vi "BNO055 Read Eular Example.vi"() -> ()   [LabVIEW 2019]
uses:
  <vilib>/myRIO/Common/Instrument Driver Framework/myRIO v1.0/UART/vis/myRIO v1.0 Close UART.vi
  <vilib>/myRIO/Common/Instrument Driver Framework/Utilities/vis/FPGA Ref Manager.vi
  <vilib>/myRIO/Common/Instrument Driver Framework/myRIO v1.0/myRIO v1.0 Reset FPGA.vi
  <vilib>/myRIO/Common/Instrument Driver Framework/myRIO v1.0/IRQ/vis/myRIO v1.0 IRQ Info FGV.vi
  <vilib>/myRIO/Common/Instrument Driver Framework/myRIO v1.0/IRQ/vis/myRIO v1.0 Timer IRQ Info FGV.vi
  <vilib>/myRIO/Common/Instrument Driver Framework/myRIO v1.0/IRQ/vis/myRIO v1.0 ISR Agent.vi
  <vilib>/myRIO/Instrument Drivers/Utilities/vis/Reset Index.vi
  <vilib>/myRIO/Common/Instrument Driver Framework/myRIO v1.0/Resource Manager/vis/myRIO v1.0 Block Write Resource Manager.vi
  BNO055_myRIO.lvlibp
  <vilib>/myRIO/Instrument Drivers/Utilities/Utilities.lvlib
panel:
  out "error out":errorcluster
  out "calProg":T1 {"MAG" scale=0.0..1.0; "ACC" scale=0.0..1.0; "GYRO" scale=0.0..1.0; "SYS" scale=0.0..1.0}
  out "Waveform Chart":T2(graph)
  in  "Stop Button":bool
  out "EularOutput [Heading, Roll, Pitch]":dbl[](array[numeric])
  out "SysStatusCode":u8[](array[numeric]) format="%.0x"
  out "Status & Error msg & Mode":string[](array[string])
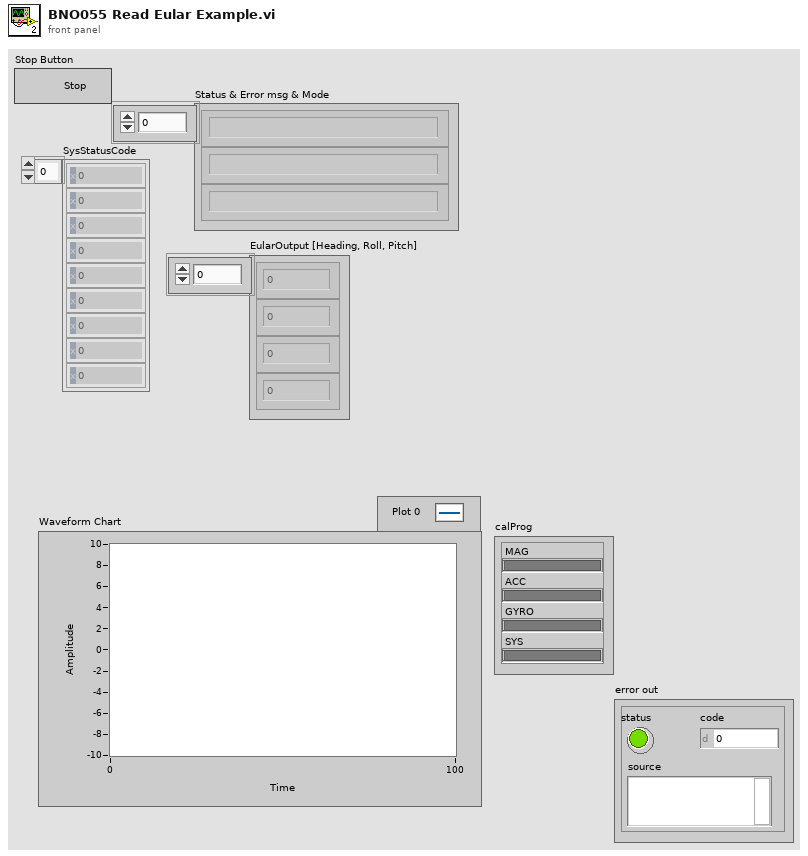
[diagram p1: front panel]
types:
  T1 = cluster{"MAG":dbl, "ACC":dbl, "GYRO":dbl, "SYS":dbl}
  T2 = cluster{"EularOutput [Heading, Roll, Pitch] [0]":dbl, "EularOutput [Heading, Roll, Pitch] [1]":dbl, "EularOutput [Heading, Roll, Pitch] [2]":dbl}
  T3 = enum16{"ConfigMode", "ACC only", "Mag only", "Gyro only", "Acc Mag", "Acc Gyro", "Mag Gyro", "AMG", "Fusion IMU", "Fusion Compass", "Fusion M4G", "NDOF_FMC_OFF", "NDOF"}
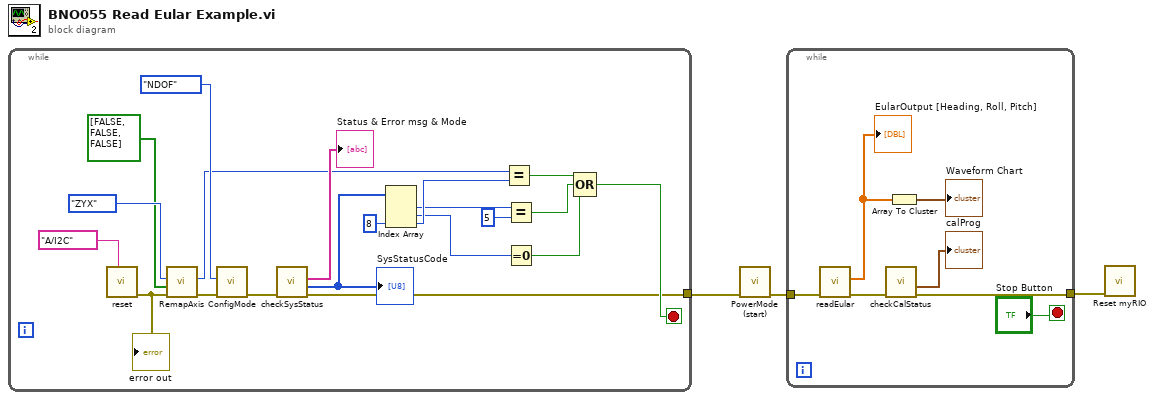
[diagram p0: block diagram]
diagram:
  n1 = while {
    tunnel: [w4] -> w3
    stop <- w5 stop-if-true
    n2 = call "reset.vi"("Channel Name"=tag "A/I2C") -> ("error out"=w22:errorcluster)  [unwired: 10 in]
    "error out" <- w22
    n3 = call "RemapAxis.vi"("error in (no error)"=w22, "AxisSign [X, Y, Z] ( F:Pos, T:Neg)"=bool[] [FALSE, FALSE, FALSE], "AxisRemap"=enum16{"XYZ", "XZY", "YXZ", "YZX", "ZXY", "ZYX"}."ZYX") -> ("Error Out"=w19:errorcluster, "hexOut"=w13:u8)  [unwired: 7 in]
    n4 = call "ConfigMode.vi"("error in (no error)"=w19, "Mode"=T3."NDOF") -> ("error out"=w17:errorcluster)  [unwired: 9 in]
    n5 = call "checkSysStatus.vi"("error in (no error)"=w17) -> ("error out"=w4:errorcluster, "SysStatusCode"=w15:u8[], "Status & Error msg & Mode"=→"Status & Error msg & Mode":string[])  [unwired: 8 in]
    "SysStatusCode" <- w15
    n6 = Index Array(array=w15, index #3=8 ("index")) -> (element #1=w10:u8, element #2=w9:u8, element #3=w12:u8)  [unwired: 2 in]
    n7 = Equal?(x=w13, y=w12) -> (x = y?=w8:bool)
    n8 = Equal?(x=w10, y=u8 5) -> (x = y?=w7:bool)
    n9 = Equal To 0?(x=w9) -> (x = 0?=w6:bool)
    n10 = Compound Arithmetic op=OR(w8, w7, w6) -> (w5:bool)
  }
  n11 = call "PowerMode (start).vi"("error in (no error)"=w3) -> ("error out"=w2:errorcluster)  [unwired: 10 in]
  n12 = while {
    tunnel: w2 -> [w30]
    tunnel: [w24] -> w1
    stop <- "Stop Button" stop-if-true
    n13 = call "readEular.vi"("error in (no error)"=w30) -> ("error out"=w29:errorcluster, "EularOutput [Heading, Roll, Pitch]"=w27:dbl[])  [unwired: 9 in]
    "EularOutput [Heading, Roll, Pitch]" <- w27
    n14 = call "checkCalStatus.vi"("error in (no error)"=w29) -> ("error out"=w24:errorcluster, "calProg"=→"calProg":T1)  [unwired: 9 in]
    n15 = Array To Cluster(array=w27) -> (cluster=→"Waveform Chart":T2)
  }
  n16 = call <vilib>:"Reset myRIO.vi"("error in (no error)"=w1) -> ()  [unwired: 10 in, 1 out]
